vi "Log Session Event.vi"(7 "Event Level":T1, 8 "error in (no error)":errorcluster, 10 "Event Data":string, 11 "SessionActor in":refnum<class "LoggedActor.lvclass">) -> (0 "error out":errorcluster, 3 "SessionActor out":refnum<class "LoggedActor.lvclass">)   [LabVIEW 2020, in "LoggedActor.lvclass"]
uses:
  <vilib>/gpm_packages/@cs/Network-interface/Source/Logged Actor/LoggedActor.lvclass
  <vilib>/gpm_packages/@cs/event-logger/Source/Composed Log/Types/Log Level.ctl
  <vilib>/gpm_packages/@cs/Network-interface/Source/Logged Actor/LoggedActor.lvclass/LoggedActor.ctl
  <vilib>/gpm_packages/@cs/event-logger/Source/Composed Log/LoggerReference/LoggerReference.lvclass/LoggerReference.ctl
  <vilib>/gpm_packages/@cs/event-logger/Source/Composed Log/LoggerReference/Log.vi
  <vilib>/gpm_packages/@cs/event-logger/Source/Composed Log/LoggerReference/Get Valid Event Time.vi
  <vilib>/gpm_packages/@cs/event-logger/Source/Composed Log/LoggerReference/Remove Stale Logs.vi
  <vilib>/gpm_packages/@cs/event-logger/Source/Composed Log/LoggerReference/LoggerReference.lvclass
  <vilib>/gpm_packages/@cs/event-logger/Source/Composed Log/Composed Log.lvlib
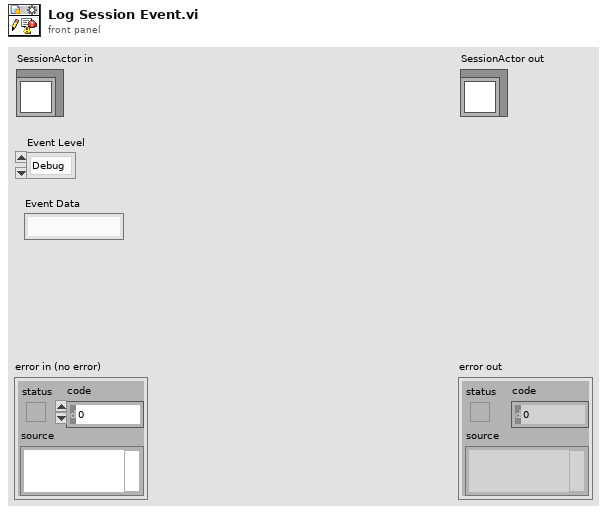
[diagram p1: front panel]
types:
  T1 = typedef "Composed Log.lvlib/Log Level.ctl" = enum16{"Debug", "Info", "Warning", "Error", "Critical"}
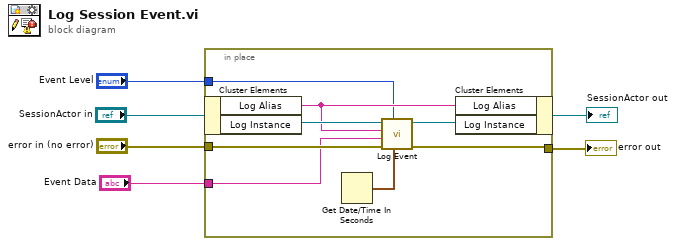
[diagram p0: block diagram]
diagram:
  n1 = in-place {
    in-place-border: "Event Level" -> [w11]
    in-place-border: "error in (no error)" -> [w9]
    in-place-border: [w8] -> w2
    in-place-border: "Event Data" -> [w7]
    n2 = in-place-cluster #1("SessionActor in") -> ("Log Alias"=w12:string, "Log Instance"=w14:refnum<class "LoggerReference.lvclass">)
    n3 = Get Date/Time In Seconds() -> (seconds since 1Jan1904=w10:timestamp)
    n4 = call <vilib>:"Log Event.vi"("Event Time"=w10, "Event Level"=w11, "error in (no error)"=w9, "Data To Log"=w7, "SourceID"=w12, "Log Instance"=w14) -> ("error out"=w8:errorcluster, "Log Instance Out"=w13:refnum<class "LoggerReference.lvclass">)  [unwired: 4 in]
    n5 = in-place-cluster #1("Log Alias"=w12, "Log Instance"=w13) -> (→"SessionActor out":refnum<class "LoggedActor.lvclass">)
  }
  "error out" <- w2
